vi "hp34401 multumetro mis example.vi"() -> ()   [LabVIEW 2012]
panel:
  in  "istruzioni":string=" INSTRUCTIONS:\r\rNormal Use:  When using subVIs that incorporate the error in/error out (or error I/O) structure, place this handler where you want to inform the user of an error, typically at the end of the I/O data path, as the last action of the program.  If the error in error? is ERROR, the handler creates a message describing the error and its source.  If the type of dialog = 1 (default), the message is displayed to the user, who can only acknowedge it.  If the type = 2, the user can acknowledge the message or abort execution; aborting a program with active I/O is not recommended.  If the type = 0, no message is displayed; this is used to process the error programmatically, and the error out cluster elements are wired to individual terminals for that reason.  \r\rOther Use:\n\r\nlocal testing.  To test the error code of a subVI or function that does not have the error I/O structure, you can wire its error code and a source string to the local error code and error source inputs.  If error in error? indicates no error and error code is not equal to 0, the local code and source are substituted for the error in values, and error? is set TRUE (ERROR)."
  out "message":string=" INSTRUCTIONS:\r\rNormal Use:  When using subVIs that incorporate the error in/error out (or error I/O) structure, place this handler where you want to inform the user of an error, typically at the end of the I/O data path, as the last action of the program.  If the error in error? is ERROR, the handler creates a message describing the error and its source.  If the type of dialog = 1 (default), the message is displayed to the user, who can only acknowedge it.  If the type = 2, the user can acknowledge the message or abort execution; aborting a program with active I/O is not recommended.  If the type = 0, no message is displayed; this is used to process the error programmatically, and the error out cluster elements are wired to individual terminals for that reason.  \r\rOther Use:\n\r\nlocal testing.  To test the error code of a subVI or function that does not have the error I/O structure, you can wire its error code and a source string to the local error code and error source inputs.  If error in error? indicates no error and error code is not equal to 0, the local code and source are substituted for the error in values, and error? is set TRUE (ERROR)."
  out "code":i32
  out "source":string
  out "status":bool
  out "error out":errorcluster
  out "Tensione":dbl format="%.8f"
  out "Stringa acquisita":string
  # "Configurazione del multimetro (conf:volt:dc)  e lettura  \ndel dato (:read?)"
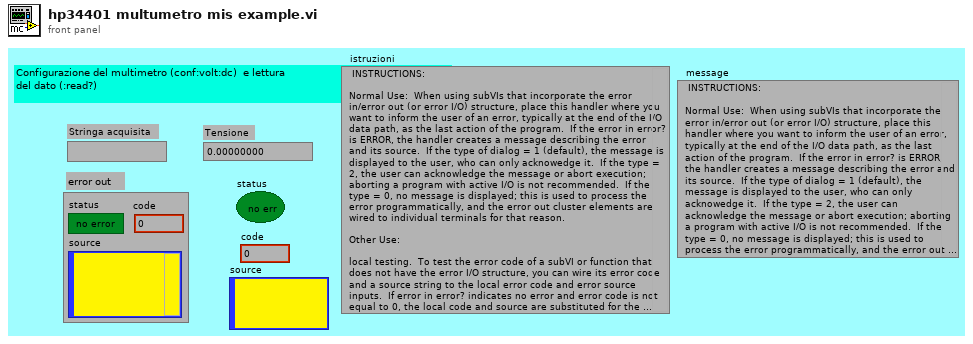
[diagram p1: front panel]
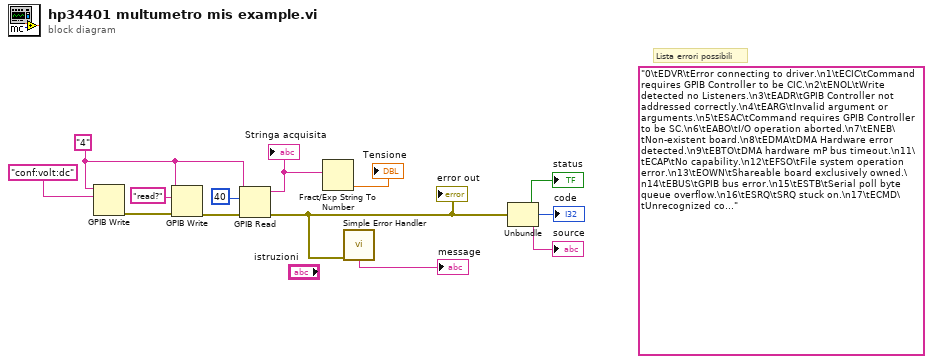
[diagram p0: block diagram]
diagram:
  (unwired) "0\tEDVR\tError connecting to driver.\n1\tECIC\tCommand requires GPIB Controller to be CIC.\n2\tENOL\tWrite detected no Listeners.\n3\tEADR\tGPIB Controller not addressed correctly.\n4\tEARG\tInvalid argument or arguments.\n5\tESAC\tCommand requires GPIB Controller to be SC.\n6\tEABO\tI/O operation aborted.\n7\tENEB\tNon-existent board.\n8\tEDMA\tDMA Hardware error detected.\n9\tEBTO\tDMA hardware mP bus timeout.\n11\tECAP\tNo capability.\n12\tEFSO\tFile system operation error.\n13\tEOWN\tShareable board exclusively owned.\n14\tEBUS\tGPIB bus error.\n15\tESTB\tSerial poll byte queue overflow.\n16\tESRQ\tSRQ stuck on.\n17\tECMD\tUnrecognized command.\n19\tEBNP\tBoard not present.\n20\tETAB\tTable error.\n30\tNADDR\tNo GPIB address input.\n31\tNSTRG\tNo string input (write).\n32\tNCNT\tNo count input (read)." ("error code")
  w10 = "4"
  # "Lista errori possibili"
  n1 = GPIB Write(0:w10, 1:"conf:volt:dc" ("reset")) -> (6:w8:errorcluster)  [unwired: 3 in, 1 out]
  n2 = GPIB Write(0:w10, 1:"read?" ("ident"), 3:w8) -> (6:w3:errorcluster)  [unwired: 2 in, 1 out]
  n3 = GPIB Read(0:w10, 1:40, 3:w3) -> (5:w4:string, 7:w1:errorcluster)  [unwired: 2 in, 1 out]
  "Stringa acquisita" <- w4
  "error out" <- w1
  n4 = Fract/Exp String To Number(string=w4) -> (number=→"Tensione":dbl)  [unwired: 3 in, 1 out]
  n5 = call <vilib>:"Simple Error Handler.vi"("error in (no error)"=w1) -> ("message"=→"message":string)  [unwired: 4 in, 4 out]
  n6 = Unbundle(w1) -> ("status"=→"status":bool, "code"=→"code":i32, "source"=→"source":string)
